vi "Get RemIO UI Ref.vi"(8 "error in (no error)":errorcluster, 11 "RemIO Module in":refnum<class "RemIO Module.lvclass">) -> (0 "error out":errorcluster, 2 "VI Refnum":refnum<vi>, 3 "RemIO Module out":refnum<class "RemIO Module.lvclass">)   [LabVIEW 2020, in "Modules.lvlib" / "RemIO Module.lvclass"]
uses:
  RemIO Module.lvclass
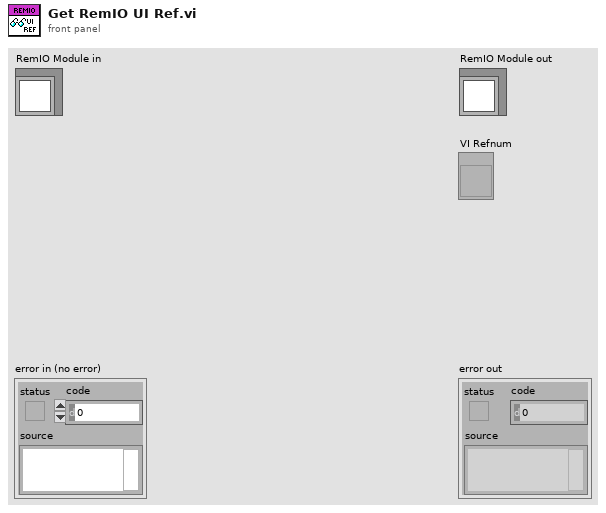
[diagram p1: front panel]
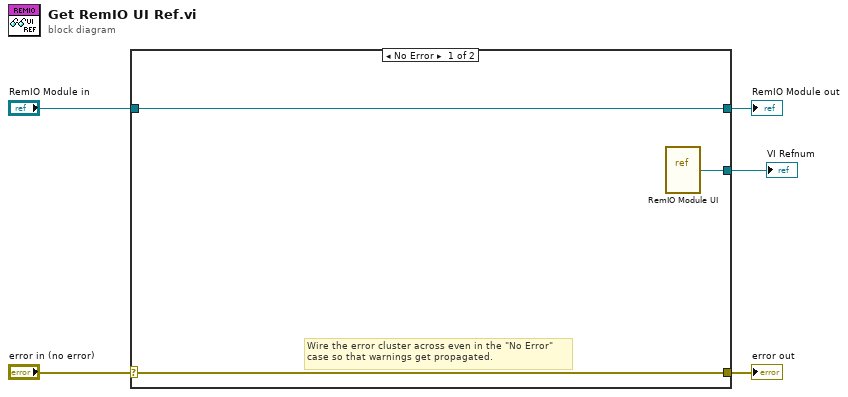
[diagram p0: block diagram]
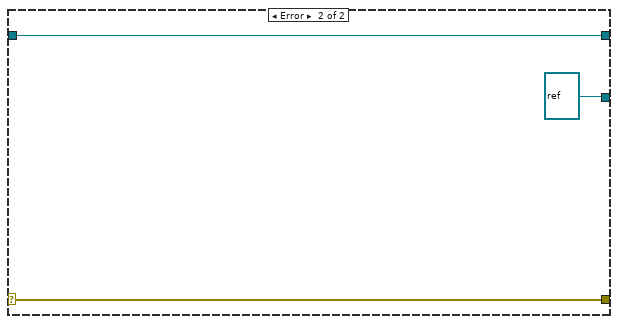
[diagram p2: hidden frame]
diagram:
  n1 = case shown="No Error" "error in (no error)" {
    selector: "error in (no error)" -> [w7 w11]
    tunnel: [w7 w11] -> w4
    tunnel: [w8 w10] -> w2
    tunnel: "RemIO Module in" -> [w8 w10]
    tunnel: [w6 refnum<vi> refnum] -> w1
    frame No Error {
      # "Wire the error cluster across even in the \"No Error\"\ncase so that warnings get propagated."
      n2 = vi-ref "RemIO Module UI.vi"() -> (w6:refnum<vi>)
    }
    frame Error {
    }
  }
  "error out" <- w4
  "RemIO Module out" <- w2
  "VI Refnum" <- w1
